vi "5_Timers.vi"() -> ()   [LabVIEW 2012]
uses:
  <userlib>/BotSpeak/VIs/Scripting/URAPI_InitTimer_num.vi
  <userlib>/BotSpeak/VIs/Scripting/URAPI_Delay_num.vi
  <userlib>/BotSpeak/VIs/Scripting/URAPI_Timer_num.vi
panel:
  out "BotSpeak":string="SET var,1\nSET TMR[1],0\nWAIT 0.2\nGET TMR[1]\nGET TMR[var]\nSET TMR[var],var\nWAIT 0.2\nGET TMR[var]\nSCRIPT\nSET TMR[2],0\nSET timer,0\nWAIT 1.000000\nSET timer,TMR[2]\nSET sum,timer\nSET more,3\nSET answer,timer\nSUB answer,1000\nend\nENDSCRIPT\nRUN&WAIT 0\nGET sum\nGET more\nGET answer\n\n"
  out "expected response":string="1\r\n0\r\n200\r\n223\r\n235\r\n1\r\n200\r\n226\r\nstart script\r\nend script\r\n.........\nDone\r\n1002\r\n3\r\n2\r\n"
  out "response":string="1\r\n0\r\n200\r\n223\r\n235\r\n1\r\n200\r\n226\r\nstart script\r\nend script\r\n.........\nDone\r\n1002\r\n3\r\n2\r\n"
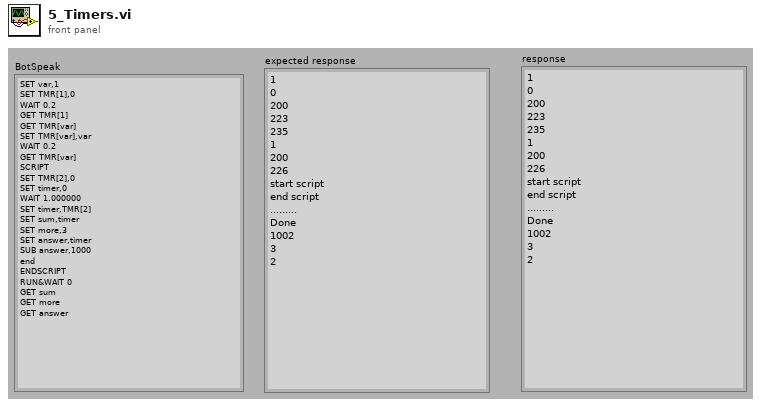
[diagram p1: front panel]
types:
  T1 = typedef "URAPI_Control.ctl" = cluster{"Script":string, "Whiles":u8[], "Ifs":u8[], "Supress Err":bool, "Errors":string}
  T2 = typedef "BotSpeak_Control.ctl" = cluster{"Address":string, "Reply EOF":string, "Hardware":path, "Retries":i8, "Timeout":i32}
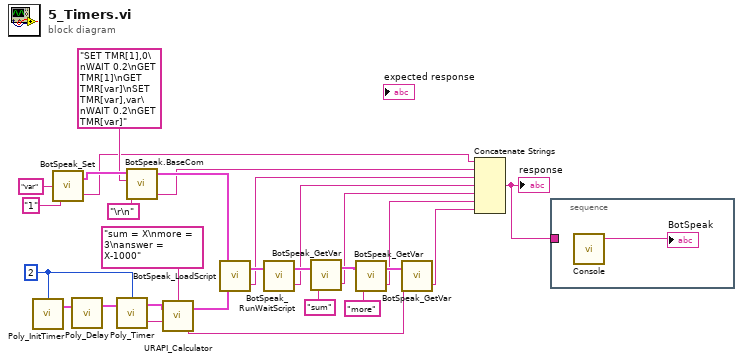
[diagram p0: block diagram]
diagram:
  w2 = u8 2 ("Timer")
  n1 = call-poly <userlib>:"Poly_InitTimer.vi"("Timer"=w2) -> ("URAPI Script out"=w6:T1)  [unwired: 3 in, 1 out]
  n2 = call <userlib>:"BotSpeak_Set.vi"("value"="1", "Variable In"="var") -> ("response"=w13:string, "Bot Settings"=w25:T2)  [unwired: 1 in]
  n3 = call-poly <userlib>:"Poly_Delay.vi"("URAPI Script"=w6) -> ("URAPI Script out"=w5:T1)  [unwired: 4 in]
  n4 = call-poly <userlib>:"Poly_Timer.vi"("URAPI Script"=w5, "Timer"=w2) -> ("Variable out"=w3:string, "URAPI Script out"=w4:T1)  [unwired: 2 in]
  n5 = call <userlib>:"BotSpeak.BaseCom.vi"("Termination"="\r\n", "command"="SET TMR[1],0\nWAIT 0.2\nGET TMR[1]\nGET TMR[var]\nSET TMR[var],var\nWAIT 0.2\nGET TMR[var]" ("String"), "Bot Settings in"=w25) -> ("response"=w12:string, "Bot Settings out"=w21:T2)  [unwired: 2 in]
  n6 = call <userlib>:"URAPI_Calculator.vi"("X"=w3, "URAPI Script"=w4, "Formula"="sum = X\nmore = 3\nanswer = X-1000") -> ("Variable Out"=w14:string, "URAPI Script"=w22:T1)  [unwired: 1 in]
  n7 = call <userlib>:"BotSpeak_LoadScript.vi"("URAPI Script"=w22, "Bot Settings"=w21) -> ("total response"=w11:string, "Bot Settings"=w20:T2)
  n8 = call <userlib>:"BotSpeak_RunWaitScript.vi"("Bot Settings"=w20) -> ("response"=w10:string, "Bot Settings"=w19:T2)  [unwired: 1 in]
  n9 = call <userlib>:"BotSpeak_GetVar.vi"("Variable In"="sum", "Bot Settings"=w19) -> ("value"=w9:string, "Bot Settings out"=w16:T2)
  n10 = call <userlib>:"BotSpeak_GetVar.vi"("Variable In"="more", "Bot Settings"=w16) -> ("value"=w8:string, "Bot Settings out"=w15:T2)
  n11 = call <userlib>:"BotSpeak_GetVar.vi"("Variable In"=w14, "Bot Settings"=w15) -> ("value"=w7:string)  [unwired: 1 out]
  n12 = Concatenate Strings(w13, w12, w11, w10, w9, w8, w7) -> (w1:string)
  "response" <- w1
  n13 = stacked-sequence {
    tunnel: w1 -> [_]
    frame #0 {
      n14 = call <userlib>:"Console.vi"() -> ("BotSpeak"=→"BotSpeak":string)  [unwired: 4 in, 1 out]
    }
  }
